vi "SR400 SetCountSource.vi"(6 "error in (no error)":errorcluster, 7 "T Source":u16(ring) caption="Source «T»" items=["10 MHz"=0, "Input 2"=2, "Trig"=3], 8 "A Source":u16(ring)=1 caption="Source «A»" items=["Input 1"=1, "10 MHz"=0], 9 "B Source":u16(ring)=2 caption="Source «B»" items=["Input 1"=1, "Input 2"=2], 10 "VISA Port In":refnum<visa-resource-name>="GPIB0::23::INSTR") -> (0 "error out":errorcluster, 3 "VISA Port Out":refnum<visa-resource-name>="GPIB0::23::INSTR")   [LabVIEW 2019]
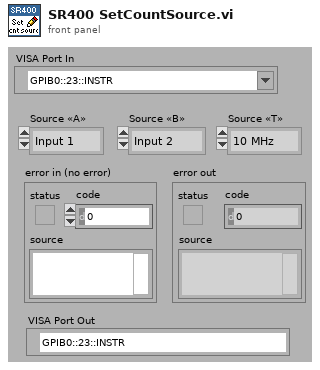
[diagram p1: front panel]
types:
  T1 = enum16{"Lit le Statut", "Configure", "Oper. incomp."}
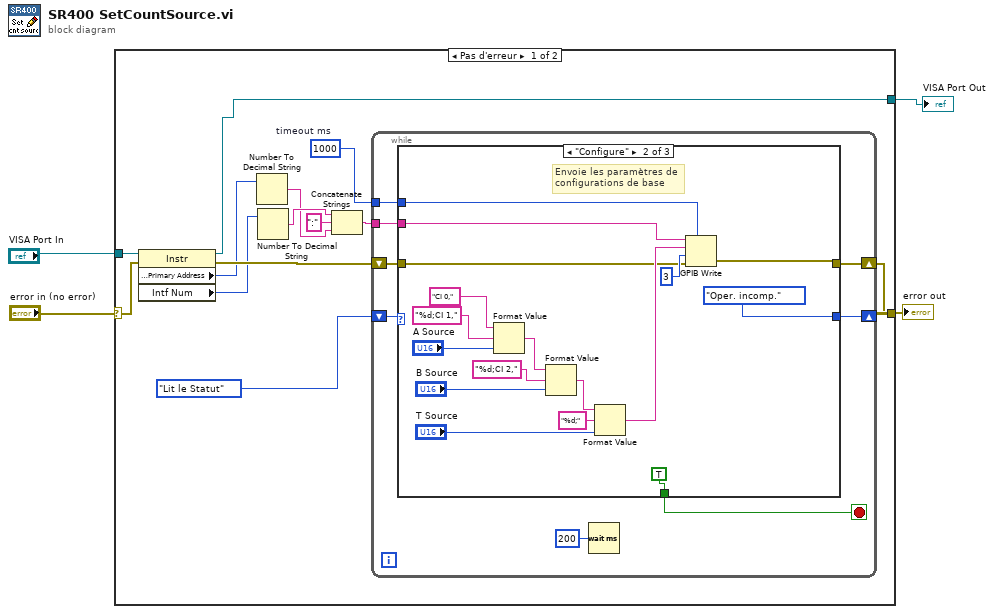
[diagram p0: block diagram]
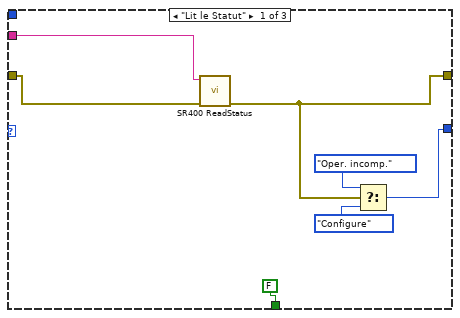
[diagram p2: hidden frame]
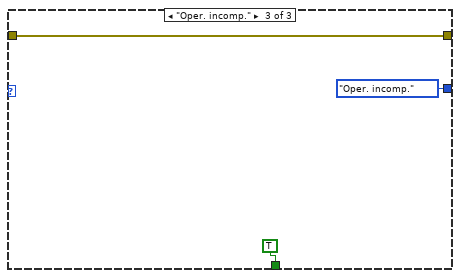
[diagram p3: hidden frame]
diagram:
  n1 = case shown="Pas d'erreur" "error in (no error)" {
    selector: "error in (no error)" -> [w17 w54]
    tunnel: [w11 w54] -> w3
    tunnel: "VISA Port In" -> [w16 w53]
    tunnel: [w5 w53] -> w1
    frame No Error {
      w12 = 1000  # timeout ms
      n2 = property class="Instr"(reference=w16, error in=w17) -> (reference out=w5:refnum<visa-resource-name>, error out=w15:errorcluster, "GPIB Settings:Primary Address"=w13:u16, "Intf Num"=w10:u16)
      n3 = Number To Decimal String(number=w13) -> (decimal integer string=w7:string)  [unwired: 1 in]
      n4 = Number To Decimal String(number=w10) -> (decimal integer string=w8:string)  [unwired: 1 in]
      n5 = Concatenate Strings(w8, ":" ("string"), w7) -> (w6:string)
      n6 = while {
        shift-right: [w19] -> _
        shift-left: T1."Lit le Statut" -> [w25]
        tunnel: w6 -> [w23]
        shift-right: [w22] -> w11
        shift-left: w15 -> [w24]
        tunnel: w12 -> [w21]
        stop <- w20 stop-if-true
        n7 = case shown="\"Configure\"" w25 {
          tunnel: w24 -> [w31 w36 w52]
          tunnel: w23 -> [w30 w35 _]
          tunnel: [w26 w33 w52] -> w22
          tunnel: w21 -> [_ w48 _]
          tunnel: [FALSE ("Configuration\neffectuée") TRUE ("Configuration\neffectuée") TRUE ("Configuration\neffectuée")] -> w20
          tunnel: [w27 T1."Oper. incomp." T1."Oper. incomp."] -> w19
          frame "Lit le Statut" {
            n8 = call <userlib>:"SR400 ReadStatus.vi"("error in"=w31, "Address string"=w30) -> ("Error Out"=w26:errorcluster)  [unwired: 6 in, 1 out]
            n9 = Select(t=T1."Oper. incomp.", s=w26, f=T1."Configure") -> (s? t:f=w27:T1)
          }
          frame "Configure" {
            # "Envoie les paramètres de configurations de base"
            n10 = Format Value(string ("")="CI 0,", format string="%d;CI 1,", value (0)="A Source") -> (output string=w44:string)
            n11 = Format Value(string ("")=w44, format string="%d;CI 2,", value (0)="B Source") -> (output string=w39:string)
            n12 = Format Value(string ("")=w39, format string="%d;", value (0)="T Source") -> (output string=w37:string)
            n13 = GPIB Write(0:w35, 1:w37, 2:i16 3 ("mode (0)"), 3:w36, 4:w48) -> (6:w33:errorcluster)  [unwired: 1 out]
          }
          frame "Oper. incomp." {
          }
        }
        n14 = Wait (ms)(milliseconds to wait=u32 200) -> ()  [unwired: 1 out]
      }
    }
    frame Error {
    }
  }
  "error out" <- w3
  "VISA Port Out" <- w1
